vi "least square linear interpolation.vi"(10 "X":dbl[](array[numeric])=[1.0, 2.0, 3.0], 11 "Y":dbl[](array[numeric])=[-1.0, -2.0, -3.0]) -> (1 "intercept":dbl=-0.0, 2 "slope":dbl=-1.0)   [LabVIEW 2015]
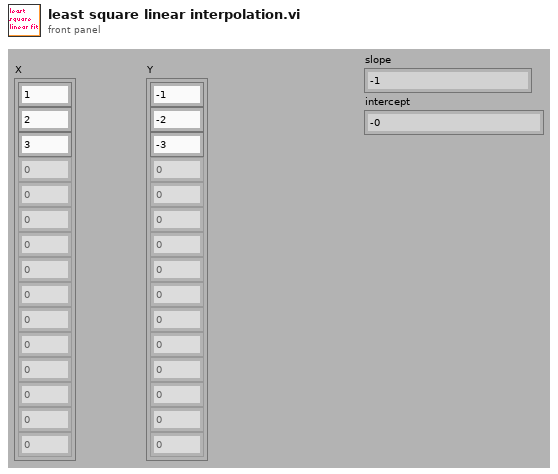
[diagram p1: front panel]
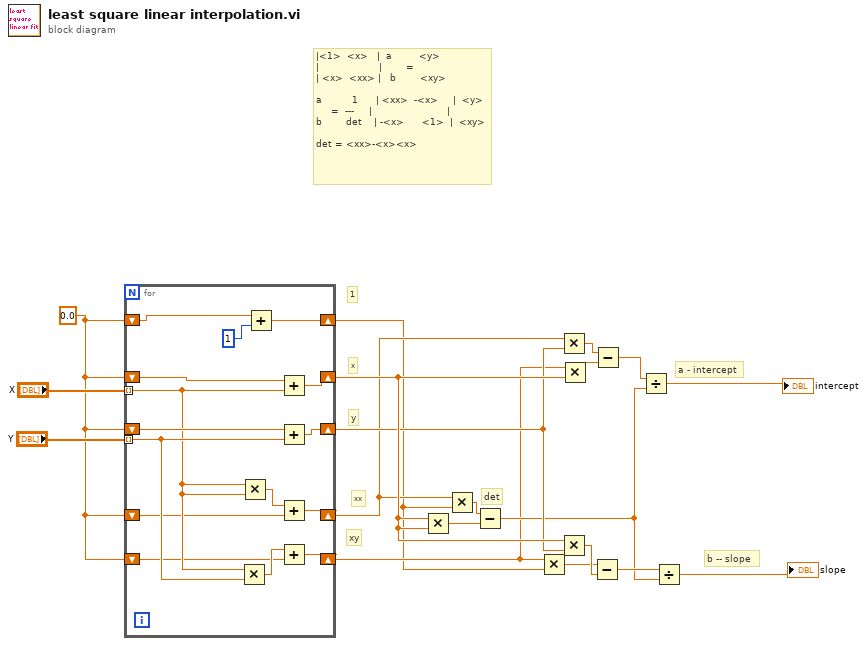
[diagram p0: block diagram]
diagram:
  w17 = 0.0
  # "b -- slope"
  # "a - intercept"
  # "|<1>  <x>   |  a         <y>\n|                    |        =   \n| <x>  <xx> |   b        <xy> \n\na          1      | <xx>  -<x>     |  <y>\n     =  ---     |                         |\nb        det    | -<x>      <1>  |  <xy>\n\ndet = <xx>-<x><x>"
  # "det"
  # "xy"
  # "xx"
  # "y"
  # "x"
  # "1"
  n1 = for {
    shift-right: [w34] -> w2
    shift-left: w17 -> [w33]
    shift-right: [w30] -> w10
    shift-left: w17 -> [w31]
    tunnel: "X" -> [w26] mode=indexing
    tunnel: "Y" -> [w27] mode=indexing
    shift-right: [w28] -> w9
    shift-left: w17 -> [w29]
    shift-right: [w22] -> w5
    shift-left: w17 -> [w23]
    shift-right: [w20] -> w3
    shift-left: w17 -> [w21]
    n2 = Multiply(x=w26, y=w27) -> (x*y=w24:dbl)
    n3 = Multiply(x=w26, y=w26) -> (x*y=w25:dbl)
    n4 = Add(x=w33, y=1) -> (x+y=w34:dbl)
    n5 = Add(x=w31, y=w26) -> (x+y=w30:dbl)
    n6 = Add(x=w29, y=w27) -> (x+y=w28:dbl)
    n7 = Add(x=w25, y=w23) -> (x+y=w22:dbl)
    n8 = Add(x=w24, y=w21) -> (x+y=w20:dbl)
  }
  n9 = Multiply(x=w10, y=w10) -> (x*y=w16:dbl)
  n10 = Multiply(x=w5, y=w2) -> (x*y=w4:dbl)
  n11 = Subtract(x=w4, y=w16) -> (x-y=w8:dbl)
  n12 = Multiply(x=w3, y=w2) -> (x*y=w1:dbl)
  n13 = Multiply(x=w5, y=w9) -> (x*y=w15:dbl)
  n14 = Multiply(x=w10, y=w9) -> (x*y=w12:dbl)
  n15 = Multiply(x=w3, y=w10) -> (x*y=w14:dbl)
  n16 = Subtract(x=w1, y=w12) -> (x-y=w11:dbl)
  n17 = Subtract(x=w15, y=w14) -> (x-y=w13:dbl)
  n18 = Divide(x=w13, y=w8) -> (x/y=→"intercept":dbl)
  n19 = Divide(x=w11, y=w8) -> (x/y=→"slope":dbl)
